vi "Parse String.vi"(7 "Paths":string[](array[string]), 8 "error in (no error)":errorcluster, 10 "String":string, 11 "YAML Parser in":refnum<class "YAML Parser.lvclass">) -> (0 "error out":errorcluster, 3 "YAML Parser out":refnum<class "YAML Parser.lvclass">)   [LabVIEW 2015, in "YAML Parser.lvclass"]
uses:
  YAML Parser.lvclass
  YAML Parser.lvclass/YAML Parser.ctl
panel:
  out "Remaining String":string
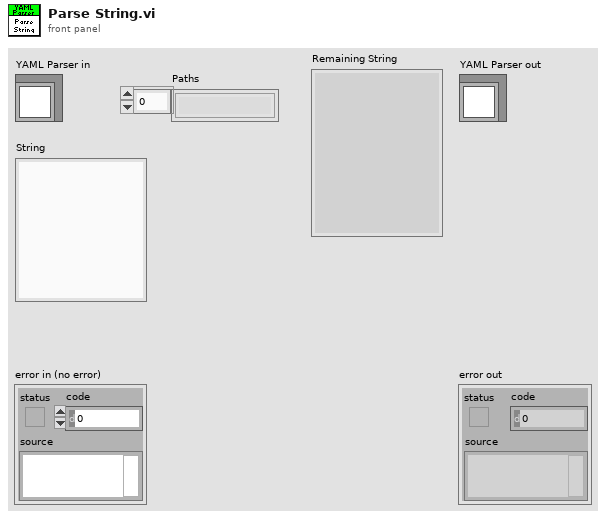
[diagram p1: front panel]
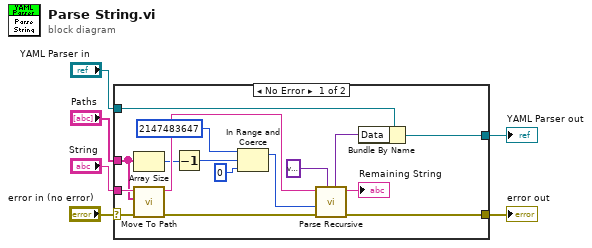
[diagram p0: block diagram]
diagram:
  n1 = case shown="No Error" "error in (no error)" {
    selector: "error in (no error)" -> [w16 w24]
    tunnel: [w19 w24] -> w5
    tunnel: [w20 w23] -> w3
    tunnel: "YAML Parser in" -> [w22 w23]
    tunnel: "String" -> [w14 _]
    tunnel: "Paths" -> [w12 _]
    frame No Error {
      n2 = Array Size(array=w12) -> (size(s)=w11:i32)
      n3 = call "Move To Path.vi"("error in (no error)"=w16, "Paths"=w12, "String"=w14) -> ("error out"=w15:errorcluster, "String out"=w13:string)  [unwired: 7 in]
      n4 = Decrement(x=w11) -> (x-1=w10:i32)
      n5 = In Range and Coerce(upper limit=2147483647, x=w10, lower limit=0) -> (coerced(x)=w8:i32)  [unwired: 1 out]
      n6 = call "Parse Recursive.vi"("Variant"=variant, "error in (no error)"=w15, "Level"=w8, "String"=w13) -> ("error out"=w19:errorcluster, "Remaining String"=→"Remaining String":string, "Variant out"=w18:variant)  [unwired: 5 in]
      n7 = Bundle By Name(cluster=w22, "Data"=w18) -> (w20:refnum<class "YAML Parser.lvclass">)
    }
    frame Error {
    }
  }
  "error out" <- w5
  "YAML Parser out" <- w3
